vi "GDSLvClass_StoreClassColors.vi"(0 "Library Refnum":refnum<vi>, 1 "LvClassIconSettings":T1={"Frame"=0, "Frame thickness"=3, "Header Background"=8453954, "Header Text"=0, "ColorPublic"=16121600, "ColorProtected"=16777215, "ColorPrivate"=16777215, "Body Text"=0, "ClassBodyIcon"=""} {"Frame thickness" min=1 max=3 step=1}, 5 "error in (no error)":errorcluster) -> (14 "Library Refnum":refnum<vi>, 19 "error out":errorcluster)   [LabVIEW 2020]
uses:
  <resource>/Framework/Providers/Open_GDS/ClassProviders/Common/LvClass_class/GDSLvClass_IconSettingsType.ctl
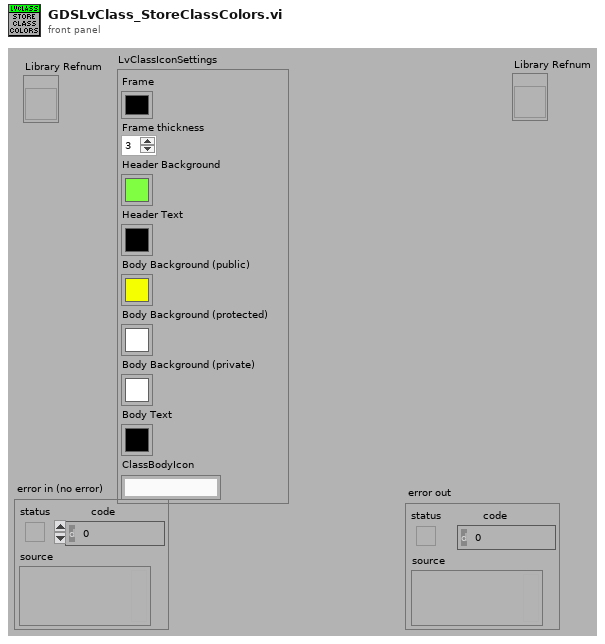
[diagram p1: front panel]
types:
  T1 = typedef "GDSLvClass_IconSettingsType.ctl" = cluster{"Frame":u32, "Frame thickness":u8, "Header Background":u32, "Header Text":u32, "ColorPublic":u32, "ColorProtected":u32, "ColorPrivate":u32, "Body Text":u32, "ClassBodyIcon":string}
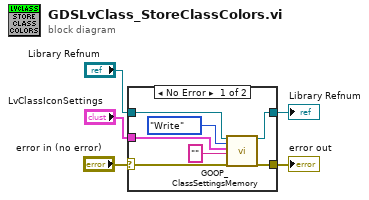
[diagram p0: block diagram]
diagram:
  n1 = case shown="No Error" "error in (no error)" {
    selector: "error in (no error)" -> [w7 w14]
    tunnel: [w8 w14] -> w4
    tunnel: "Library Refnum" -> [w12 w13]
    tunnel: [w6 w13] -> w2
    tunnel: "LvClassIconSettings" -> [w10 _]
    frame No Error {
      n2 = call <resource>:"GOOP_ClassSettingsMemory.vi"("Library Refnum"=w12, "Action"=enum16{"Read", "Write"}."Write", "LvClassIconSettingsIn"=w10, "ItemIconIn"="", "error in"=w7) -> ("Library Refnum"=w6:refnum<vi>, "error out"=w8:errorcluster)  [unwired: 9 in, 4 out]
    }
    frame Error {
    }
  }
  "Library Refnum" <- w2
  "error out" <- w4
